vi "Replace Class Inputs.vi"(8 "Error In":errorcluster, 9 "Target VI Path":path, 10 "Target Class Path":path, 11 "Template VI Path":path) -> (0 "Error Out":errorcluster, 3 "VI Ref out":refnum<vi>)   [LabVIEW 2013, in "Scripter.lvlib"]
uses:
  Scripter.lvlib
  <vilib>/Utility/traverseref.llb/TRef TravTarget.ctl
  <vilib>/Utility/traverseref.llb/VI Scripting - Traverse.lvlib
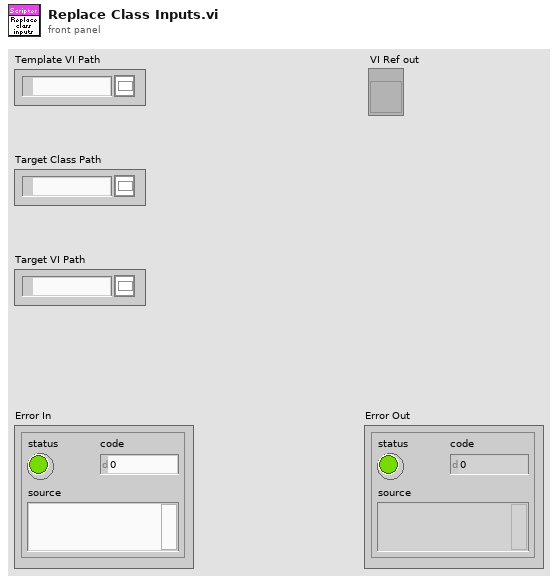
[diagram p1: front panel]
types:
  T1 = typedef "TRef TravTarget.ctl" = enum16{"FP", "BD", "Other"}
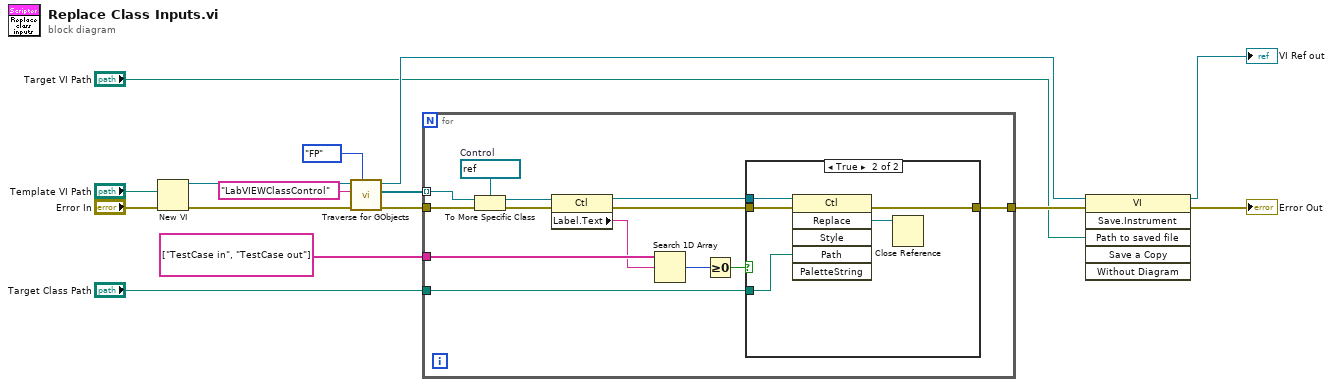
[diagram p0: block diagram]
diagram:
  n1 = New VI(8:"Error In", 10:"Template VI Path") -> (0:w13:errorcluster, 3:w6:refnum<vi>)  [unwired: 5 in]
  n2 = call <vilib>:"Traverse for GObjects.vi"("Traverse Target"=TRef_TravTarget."FP", "error in (no error)"=w13, "Class Name"="LabVIEWClassControl", "VI Refnum"=w6) -> ("error out"=w8:errorcluster, "References"=w10:refnum<vi>[], "dup VI Refnum"=w3:refnum<vi>)  [unwired: 4 in, 1 out]
  n3 = for {
    tunnel: w10 -> [w28] mode=indexing
    tunnel: string[] ["TestCase in", "TestCase out"] -> [w25]
    tunnel: w8 -> [w23]
    tunnel: "Target Class Path" -> [w18]
    tunnel: [w16] -> w5
    w26 = refnum<vi> refnum  # Control
    n4 = To More Specific Class(target class=w26, reference=w28, error in=w23) -> (specific class reference=w27:refnum<vi>, error out=w22:errorcluster)
    n5 = property class="Ctl"(reference=w27, error in=w22) -> (reference out=w20:refnum<vi>, error out=w17:errorcluster, "Label.Text"=w24:string)
    n6 = Search 1D Array(1D array=w25, element=w24) -> (index of element=w21:i32)  [unwired: 1 in]
    n7 = Greater Or Equal To 0?(x=w21) -> (x >= 0?=w19:bool)
    n8 = case shown="True" w19 {
      tunnel: w20 -> [_ w34]
      tunnel: w18 -> [_ w33]
      tunnel: w17 -> [w29 w31]
      tunnel: [w29 w30] -> w16
      frame False {
      }
      frame True {
        n9 = invoke class="Ctl" method="Replace"(reference=w34, error in=w31, "Path"=w33) -> (error out=w30:errorcluster, "Replace"=w32:refnum<vi>)  [unwired: 3 in, 4 out]
        n10 = Close Reference(reference=w32) -> ()  [unwired: 1 in, 1 out]
      }
    }
  }
  n11 = invoke class="VI" method="Save.Instrument"(reference=w3, error in=w5, "Path to saved file"="Target VI Path") -> (reference out=→"VI Ref out":refnum<vi>, error out=→"Error Out":errorcluster)  [unwired: 3 in, 4 out]
